vi "_Veritech_LVCM_Provider_LoadComplete.vi"(11 "Project":refnum<vi>) -> ()   [LabVIEW 2014]
uses:
  Support/Framework/GCMConfigurationManager/GCMConfigurationManager.lvclass
panel:
  out "error out":errorcluster
  in  "error in (no error)":errorcluster
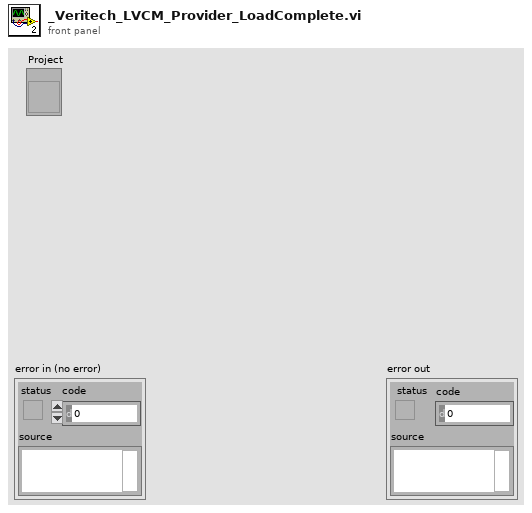
[diagram p1: front panel]
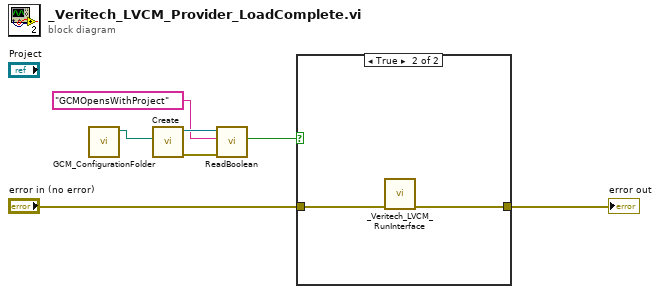
[diagram p0: block diagram]
diagram:
  n1 = call "GCM_ConfigurationFolder.vi"() -> ("ConfigurationFolder"=w3:path)  [unwired: 11 in]
  n2 = call "Create.vi"("ConfigurationFolder"=w3) -> ("error out"=w4:errorcluster, "GCMConfigurationManager out"=w5:refnum<class "GCMConfigurationManager.lvclass">)  [unwired: 9 in]
  n3 = call "ReadBoolean.vi"("error in (no error)"=w4, "Key"="GCMOpensWithProject", "GCMConfigurationManager in"=w5) -> ("Value"=w1:bool)  [unwired: 6 in, 2 out]
  n4 = case shown="True" w1 {
    tunnel: "error in (no error)" -> [w8 w10]
    tunnel: [w8 w9] -> w6
    frame False {
    }
    frame True {
      n5 = call "_Veritech_LVCM_RunInterface.vi"("error in (no error)"=w10) -> ("error out"=w9:errorcluster)  [unwired: 10 in]
    }
  }
  "error out" <- w6
